vi "ICR_Setup_SequenceLoop.vi"(8 "error in (no error)":errorcluster, 9 "QMH UI Cluster":variant, 11 "QMH ICR Cluster":T1) -> (0 "error out":errorcluster, 3 "QMH ICR Cluster":T1)   [LabVIEW 2024]
doc: "This VI updates the indicators of the ICR panel according to the parameters setup by the user and the controls in the UI main panel.\n\n1. The indicators are passed by reference through the QMH ICR Cluster.\n2. Their values are updated with the QMH UI Cluster parameters.\n3. The QMH ICR Cluster given in output contains the updated indicators."
uses:
  controls/QMH_ICR_Cluster.ctl
  controls/HARDWARE_Resources.ctl
  controls/PROCESSING_Inputs.ctl
  controls/LOOPS_Inputs.ctl
  controls/OPO_Inputs.ctl
  controls/QMH_UI_Cluster.ctl
  controls/QMH_UI_References.ctl
  controls/QMH_UI_Report.ctl
  controls/QMH_UI_Command.ctl
  controls/QMH_ICR_Command.ctl
  controls/QMH_Status.ctl
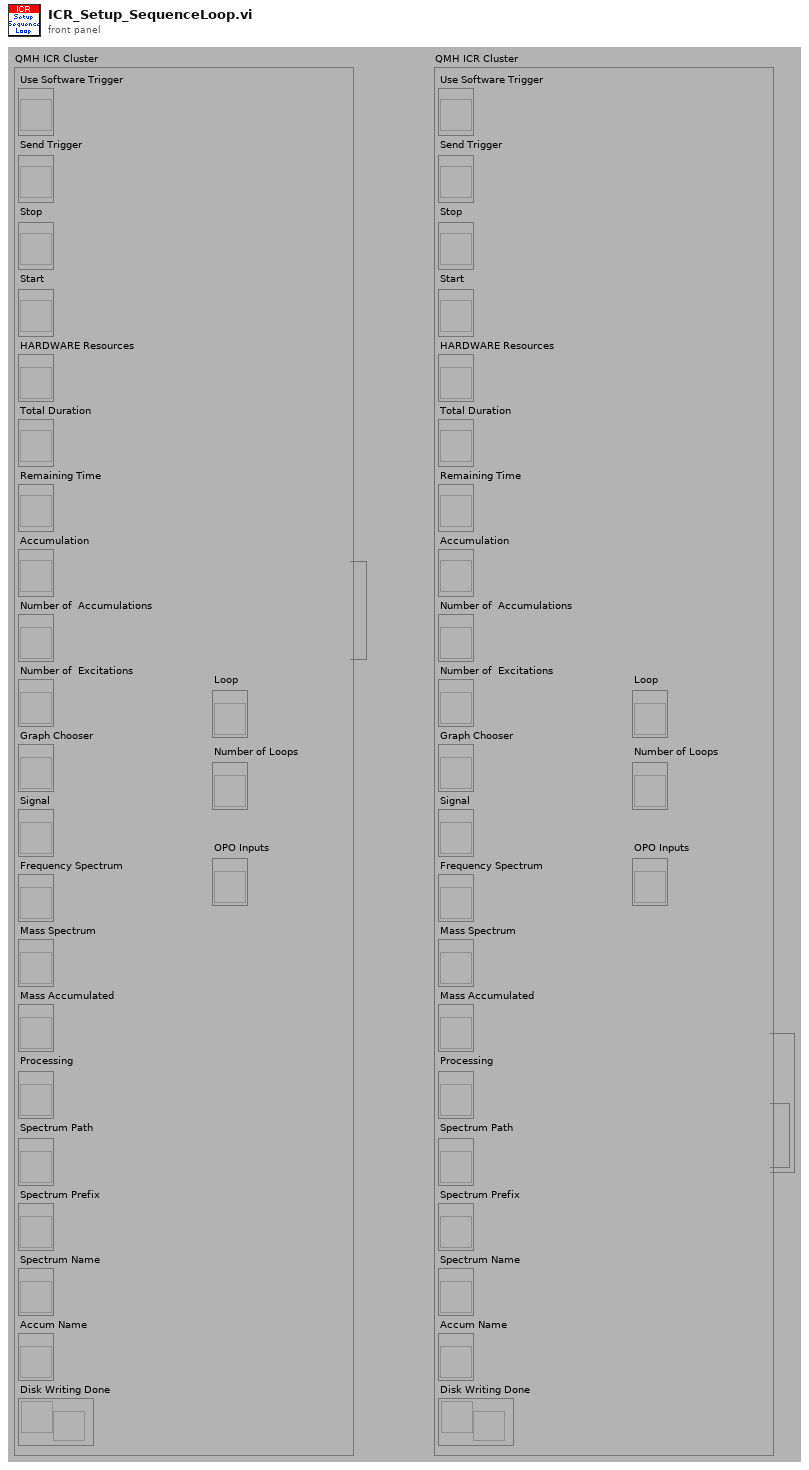
[diagram p1: front panel]
types:
  T1 = typedef "QMH_ICR_Cluster.ctl" = cluster{"Use Software Trigger":refnum<vi>, "Send Trigger":refnum<vi>, "Stop":refnum<vi>, "Start":refnum<vi>, "HARDWARE Resources":refnum<vi>, "Total Duration":refnum<vi>, "Remaining Time":refnum<vi>, "Accumulation":refnum<vi>, "Number of  Accumulations":refnum<vi>, "Number of  Excitations":refnum<vi>, "Graph Chooser":refnum<vi>, "Signal":refnum<vi>, "Frequency Spectrum":refnum<vi>, "Mass Spectrum":refnum<vi>, "Mass Accumulated":refnum<vi>, "Processing":refnum<vi>, "Spectrum Path":refnum<vi>, "Spectrum Prefix":refnum<vi>, "Spectrum Name":refnum<vi>, "Accum Name":refnum<vi>, "Disk Writing Done":refnum<notifier>, "Loop":refnum<vi>, "Number of Loops":refnum<vi>, "OPO Inputs":refnum<vi>}
  T2 = typedef "LOOPS_Inputs.ctl" = cluster{"Number of Loops":i16, "Loop Current Value":i16, "OPO Inputs":T3}
  T3 = typedef "OPO_Inputs.ctl" = cluster{"OPO AutoAlignment ON":bool, "OPO Start Value":dbl, "OPO Stop Value":dbl, "OPO Step":dbl}
  T4 = typedef "QMH_UI_Cluster.ctl" = cluster{"QMH UI References":T5, "QMH UI Report":T6}
  T5 = typedef "QMH_UI_References.ctl" = cluster{"Refnum Load":refnum<vi>, "Refnum Save As":refnum<vi>, "Refnum Start":refnum<vi>, "Refnum Exit":refnum<vi>, "Refnum Tabs":refnum<vi>, "Refnum SPECTRUM":refnum<vi>, "Refnum EXPERIMENT":refnum<vi>, "Refnum VOLTAGES":refnum<vi>, "Refnum SEQUENCE":refnum<vi>, "Refnum EXPERT":refnum<vi>, "Refnum LOOPS":refnum<vi>, "Refnum EXCIT Table":refnum<vi>, "Refnum TIMING Table":refnum<vi>, "Refnum CHANGE Experiment":refnum<vi>, "Refnum CHANGE Voltages":refnum<vi>, "Refnum CHANGE Sequence":refnum<vi>, "Refnum CHANGE Expert":refnum<vi>, "Refnum CHANGE Loops":refnum<vi>, "Refnum CHANGE Scientist":refnum<vi>, "Refnum PIL Status":refnum<vi>}
  T6 = typedef "QMH_UI_Report.ctl" = cluster{"UI Status":T7, "ICR Status":T8, "QMH Status":T9}
  T7 = typedef "QMH_UI_Command.ctl" = enum16{"Initialize", "UI Load", "UI Save", "UI Save As", "UI Change Experiment", "UI Change Voltages", "UI Change Sequence", "UI Change Expert", "UI Change Loops", "UI Change Scientist", "Ready to Start", "UI Start", "Waiting for ICR", "UI Exit", "Update Experiment", "Update Report", "Update ICR Status", "Waiting for User"}
  T8 = typedef "QMH_ICR_Command.ctl" = enum16{"Initialize", "Sequence Loop Setup", "Sequence Setup", "ICR Start", "ICR Stop", "Hardware Setup", "Next Sequence Loop", "Next Accumulation", "Waiting for Trigger", "Sequence Started", "Sequence Finished", "Sequence Loop Done", "Writing Data", "Hardware Reset", "Exit"}
  T9 = typedef "QMH_Status.ctl" = enum16{"Init", "Loading", "Setup", "Ready to Start", "Started", "Idle"}
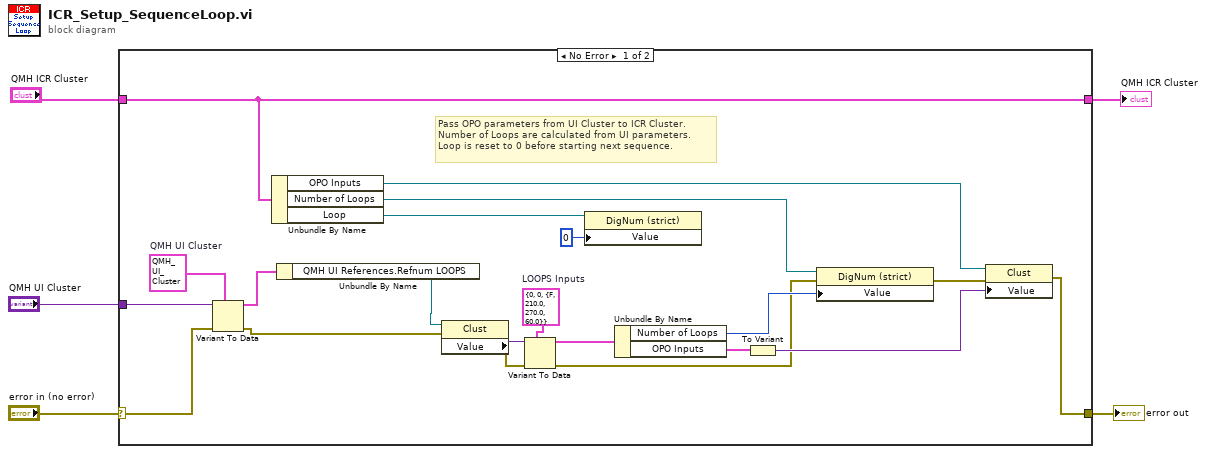
[diagram p0: block diagram]
diagram:
  n1 = case shown="No Error" "error in (no error)" {
    selector: "error in (no error)" -> [w16 w28]
    tunnel: [w9 w28] -> w5
    tunnel: "QMH UI Cluster" -> [w18 _]
    tunnel: "QMH ICR Cluster" -> [w20 w27]
    tunnel: [w20 w27] -> w1
    frame No Error {
      w24 = T2 {"Number of Loops"=0, "Loop Current Value"=0, "OPO Inputs"={"OPO AutoAlignment ON"=FALSE, "OPO Start Value"=210.0, "OPO Stop Value"=270.0, "OPO Step"=60.0}}  # LOOPS Inputs
      w26 = T4 {"QMH UI References"={"Refnum Load"=refnum, "Refnum Save As"=refnum, "Refnum Start"=refnum, "Refnum Exit"=refnum, "Refnum Tabs"=refnum, "Refnum SPECTRUM"=refnum, "Refnum EXPERIMENT"=refnum, "Refnum VOLTAGES"=refnum, "Refnum SEQUENCE"=refnum, "Refnum EXPERT"=refnum, "Refnum LOOPS"=refnum, "Refnum EXCIT Table"=refnum, "Refnum TIMING Table"=refnum, "Refnum CHANGE Experiment"=refnum, "Refnum CHANGE Voltages"=refnum, "Refnum CHANGE Sequence"=refnum, "Refnum CHANGE Expert"=refnum, "Refnum CHANGE Loops"=refnum, "Refnum CHANGE Scientist"=refnum, "Refnum PIL Status"=refnum}, "QMH UI Report"={"UI Status"=enum."Initialize", "ICR Status"=enum."Initialize", "QMH Status"=enum."Init"}}  # QMH UI Cluster
      # "Pass OPO parameters from UI Cluster to ICR Cluster.\nNumber of Loops are calculated from UI parameters.\nLoop is reset to 0 before starting next sequence."
      n2 = Variant To Data(error in=w16, type=w26, Variant=w18) -> (data=w17:T4, error out=w19:errorcluster)
      n3 = Unbundle By Name(w20) -> ("OPO Inputs"=w12:refnum<vi>, "Number of Loops"=w8:refnum<vi>, "Loop"=w7:refnum<vi>)
      n4 = Unbundle By Name(w17) -> ("QMH UI References.Refnum LOOPS"=w22:refnum<vi>)
      n5 = property class="Clust"(reference=w22, error in=w19) -> (error out=w25:errorcluster, "Value"=w23:variant)  [unwired: 1 out]
      n6 = Variant To Data(error in=w25, type=w24, Variant=w23) -> (data=w21:T2, error out=w11:errorcluster)
      n7 = property class="DigNum (strict)"(reference=w7, "Value"=i16 0) -> ()  [unwired: 1 in, 2 out]
      n8 = Unbundle By Name(w21) -> ("Number of Loops"=w15:i16, "OPO Inputs"=w14:T3)
      n9 = To Variant(anything=w14) -> (Variant=w13:variant)
      n10 = property class="DigNum (strict)"(reference=w8, error in=w11, "Value"=w15) -> (error out=w10:errorcluster)  [unwired: 1 out]
      n11 = property class="Clust"(reference=w12, error in=w10, "Value"=w13) -> (error out=w9:errorcluster)  [unwired: 1 out]
    }
    frame Error {
    }
  }
  "error out" <- w5
  "QMH ICR Cluster" <- w1
